vi "CreateMeasuresNode.vi"(7 "DOM Document":refnum<k20>, 8 "Error In":errorcluster, 11 "Measures":T1[](array[typedef]) {"Count" min=1 step=1}) -> (0 "Error Out":errorcluster, 3 "Measures Node":refnum<k20>)   [LabVIEW 2012]
uses:
  MeasureConfiguration.ctl
  libs/LV-Utilities/LV-Utilities.lvlib
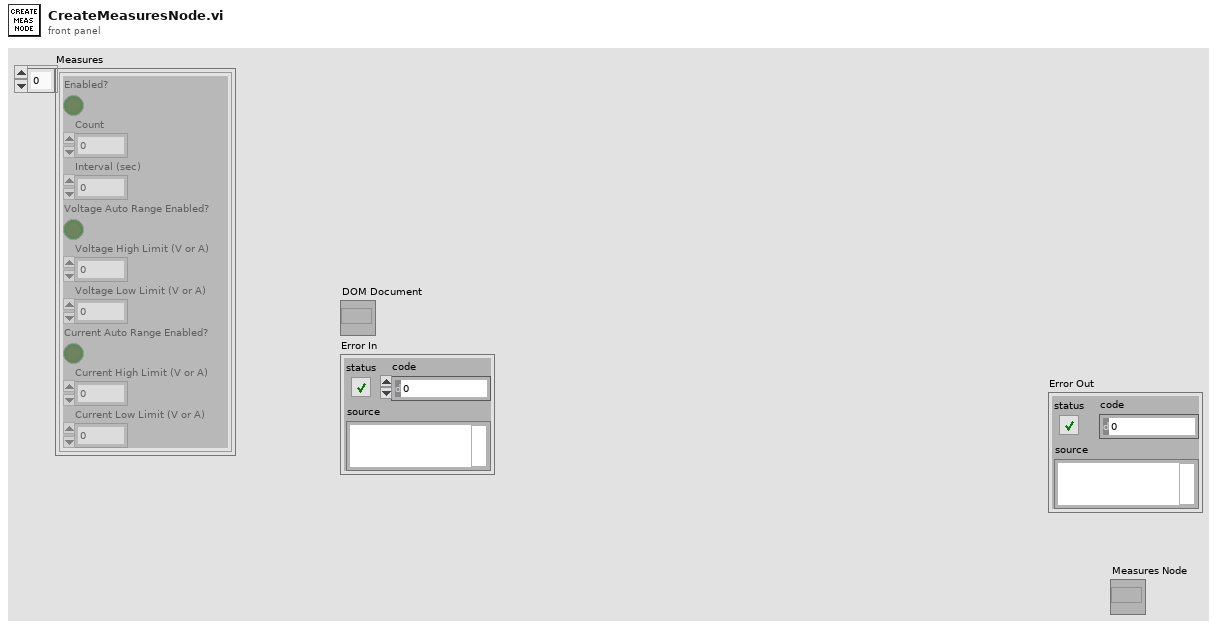
[diagram p1: front panel]
types:
  T1 = typedef "MeasureConfiguration.ctl" = cluster{"Enabled?":bool, "Count":u8, "Interval (sec)":dbl, "Voltage Auto Range Enabled?":bool, "Voltage High Limit (V or A)":dbl, "Voltage Low Limit (V or A)":dbl, "Current Auto Range Enabled?":bool, "Current High Limit (V or A)":dbl, "Current Low Limit (V or A)":dbl}
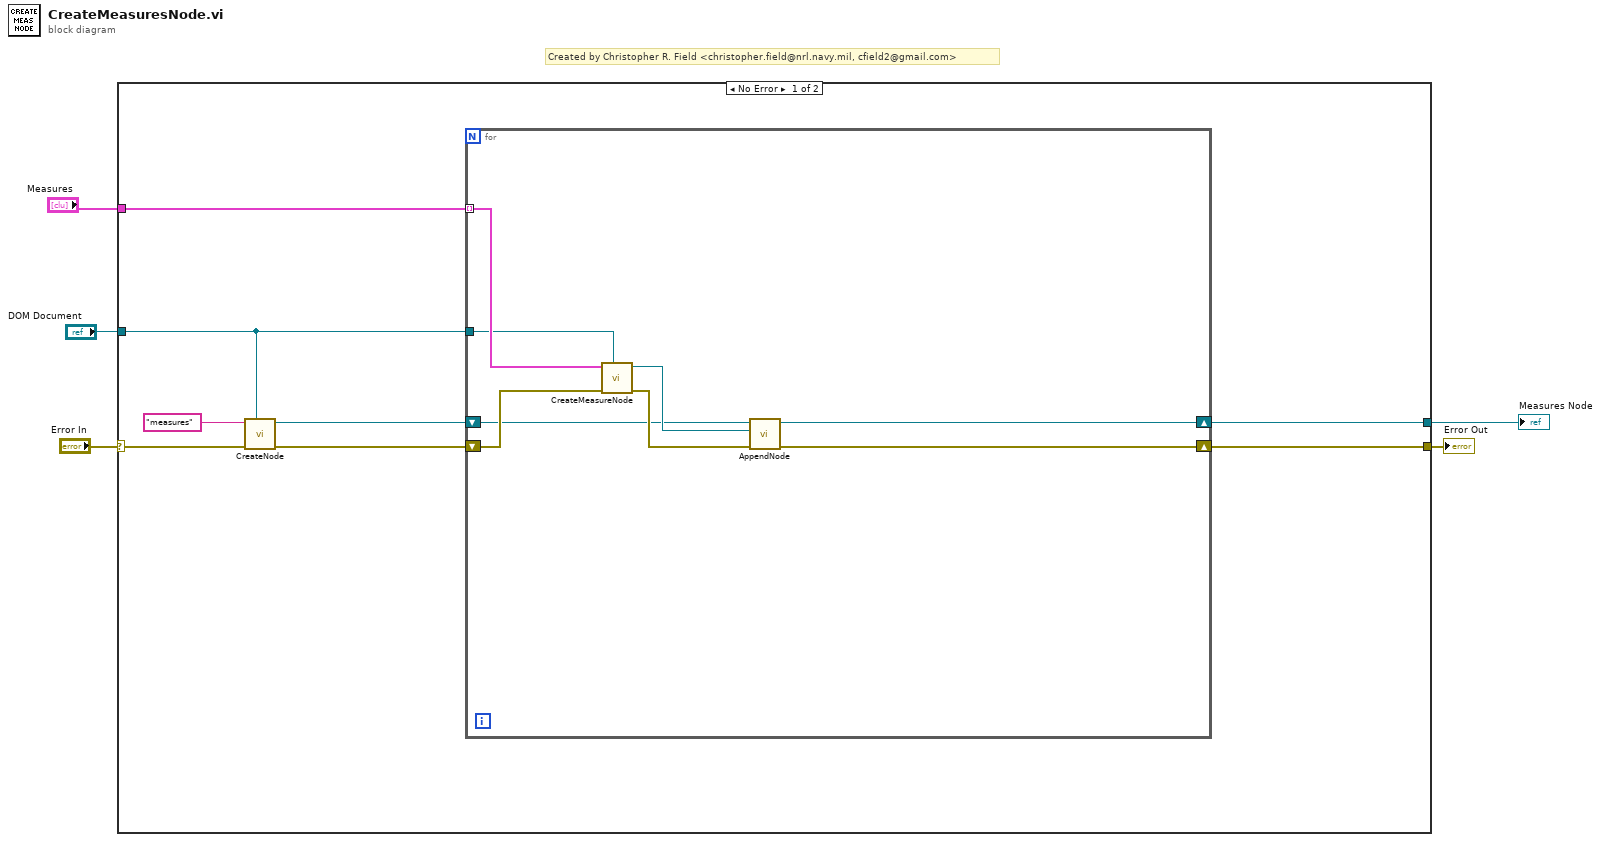
[diagram p0: block diagram]
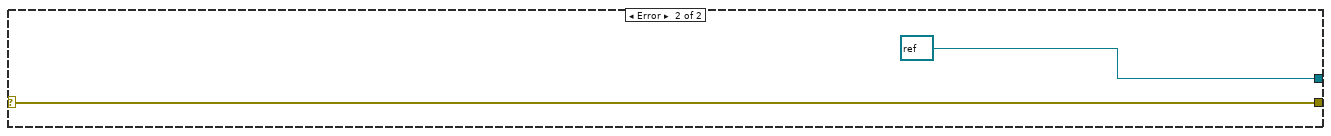
[diagram p2: hidden frame]
diagram:
  # "Created by Christopher R. Field <christopher.field@nrl.navy.mil, cfield2@gmail.com>"
  n1 = case shown="No Error" "Error In" {
    selector: "Error In" -> [w9 w23]
    tunnel: "DOM Document" -> [w6 _]
    tunnel: [w13 w23] -> w3
    tunnel: [w12 refnum<k20> refnum ("DUT Node 2")] -> w2
    tunnel: "Measures" -> [w11 _]
    frame No Error {
      n2 = call "CreateNode.vi"("DOM Document"=w6, "Error In"=w9, "Tag Name"="measures") -> ("Error out"=w8:errorcluster, "Node"=w7:refnum<k20>)  [unwired: 7 in]
      n3 = for {
        tunnel: w11 -> [w17] mode=indexing
        shift-right: [w19] -> w13
        shift-left: w8 -> [w21]
        shift-right: [w18] -> w12
        shift-left: w7 -> [w14]
        tunnel: w6 -> [w16]
        n4 = call "CreateMeasureNode.vi"("DOM Document"=w16, "Error In"=w21, "Measure Configuration"=w17) -> ("Error Out"=w20:errorcluster, "Measure Node"=w15:refnum<k20>)  [unwired: 7 in]
        n5 = call "AppendNode.vi"("Error In"=w20, "Child Node"=w15, "Parent Node In"=w14) -> ("Error Out"=w19:errorcluster, "Parent Node Out"=w18:refnum<k20>)  [unwired: 7 in]
      }
    }
    frame Error {
    }
  }
  "Error Out" <- w3
  "Measures Node" <- w2
